vi "WHH Gamma Formula.vi"(4 "data":variant, 5 "x":dbl) -> (2 "WHH(x)":dbl format="%.19f")   [LabVIEW 2021]
uses:
  WHH Formula Data.ctl
  <vilib>/gmath/NI_Gmath.lvlib
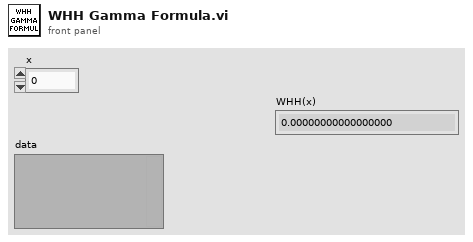
[diagram p1: front panel]
types:
  T1 = typedef "WHH Formula Data.ctl" = cluster{"t":dbl, "alpha_Maki":dbl, "lambda_SO":dbl}
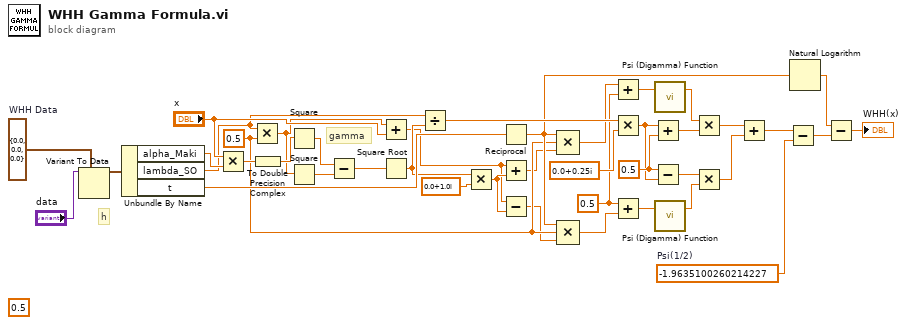
[diagram p0: block diagram]
diagram:
  w13 = 0.5
  w16 = 0.5
  (unwired) 0.5
  w36 = -1.9635100260214227  # Psi(1/2)
  w10 = 0.5
  w40 = T1 {"t"=0.0, "alpha_Maki"=0.0, "lambda_SO"=0.0}  # WHH Data
  # "gamma"
  # "h"
  n1 = Variant To Data(type=w40, Variant="data") -> (data=w38:T1)  [unwired: 1 in, 1 out]
  n2 = Unbundle By Name(w38) -> ("alpha_Maki"=w33:dbl, "lambda_SO"=w26:dbl, "t"=w37:dbl)
  n3 = Multiply(x="x", y=w33) -> (x*y=w31:dbl)
  n4 = Multiply(x=w26, y=w10) -> (x*y=w22:dbl)
  n5 = To Double Precision Complex(1:w31) -> (0:w27:cdb)
  n6 = Square(x=w27) -> (x^2=w30:cdb)
  n7 = Square(x=w22) -> (x^2=w29:dbl)
  n8 = Subtract(x=w30, y=w29) -> (x-y=w28:cdb)
  n9 = Add(x=w22, y="x") -> (x+y=w6:dbl)
  n10 = Square Root(x=w28) -> (sqrt(x)=w20:cdb)
  n11 = Divide(x=w26, y=w20) -> (x/y=w25:cdb)
  n12 = Multiply(x=w20, y=cdb 0.0+1.0i) -> (x*y=w7:cdb)
  n13 = Reciprocal(x=w37) -> (1/x=w11:dbl)
  n14 = Add(x=w6, y=w7) -> (x+y=w9:cdb)
  n15 = Subtract(x=w6, y=w7) -> (x-y=w8:cdb)
  n16 = Compound Arithmetic op=MULTIPLY(w11, w10, w9) -> (w12:cdb)
  n17 = Compound Arithmetic op=MULTIPLY(w11, w10, w8) -> (w5:cdb)
  n18 = Add(x=w12, y=w13) -> (x+y=w23:cdb)
  n19 = Multiply(x=w25, y=cdb 0.0+0.25i) -> (x*y=w15:cdb)
  n20 = Add(x=w13, y=w5) -> (x+y=w14:cdb)
  n21 = Add(x=w15, y=w16) -> (x+y=w19:cdb)
  n22 = Subtract(x=w16, y=w15) -> (x-y=w3:cdb)
  n23 = call <vilib>:"Psi (Digamma) Function.vi"("x"=w23) -> ("y(x)"=w18:dbl)  [unwired: 2 in]
  n24 = call <vilib>:"Psi (Digamma) Function.vi"("x"=w14) -> ("y(x)"=w4:dbl)  [unwired: 2 in]
  n25 = Multiply(x=w18, y=w19) -> (x*y=w17:cdb)
  n26 = Multiply(x=w3, y=w4) -> (x*y=w1:cdb)
  n27 = Add(x=w17, y=w1) -> (x+y=w2:cdb)
  n28 = Subtract(x=w2, y=w36) -> (x-y=w34:cdb)
  n29 = Natural Logarithm(1:w11) -> (0:w35:dbl)
  n30 = Subtract(x=w35, y=w34) -> (x-y=→"WHH(x)":cdb)
